vi "ToggleAqcuisitionRunning.vi"(8 "error in (no error)":errorcluster, 10 "Acquisition running":bool, 11 "ScopeBase In":refnum<class "ScopeBase.lvclass">) -> (0 "error out":errorcluster, 3 "ScopeBase Out":refnum<class "ScopeBase.lvclass">)   [LabVIEW 2025, in "ScopeBase.lvclass"]
uses:
  ScopeBase.lvclass
  ScopeBase.lvclass/ScopeBase.ctl
  <vilib>/Utility/error.llb/Error Cluster From Error Code.vi
  <vilib>/rvi/errors/niLvFpgaAdjustHostInterfaceError.vi
  <vilib>/rvi/interface/nirviReadWriteControl/nirviReadWriteControl.xnode
  FpgaRef/FpgaRefBase/Common FPGA ref.ctl
  FpgaRef/FpgaRefBase/FpgaRefBase.lvclass
  NiFpgaLv.dll
  <vilib>/rvi/interface/Simulation/niFpgaSimulationCallBeginRW.vi
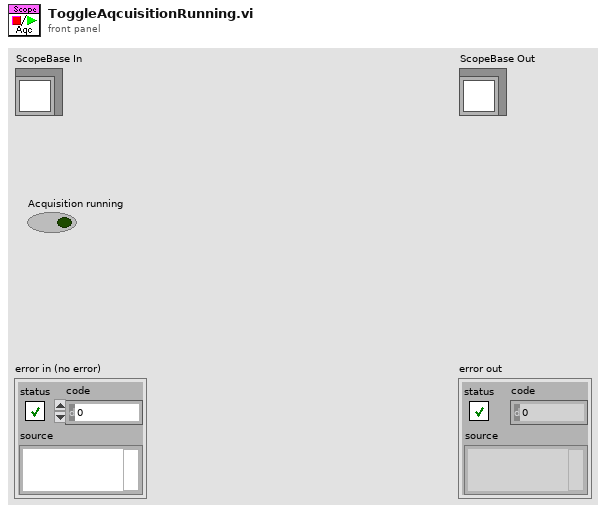
[diagram p1: front panel]
types:
  T1 = typedef "Common FPGA ref.ctl" = refnum<k20>
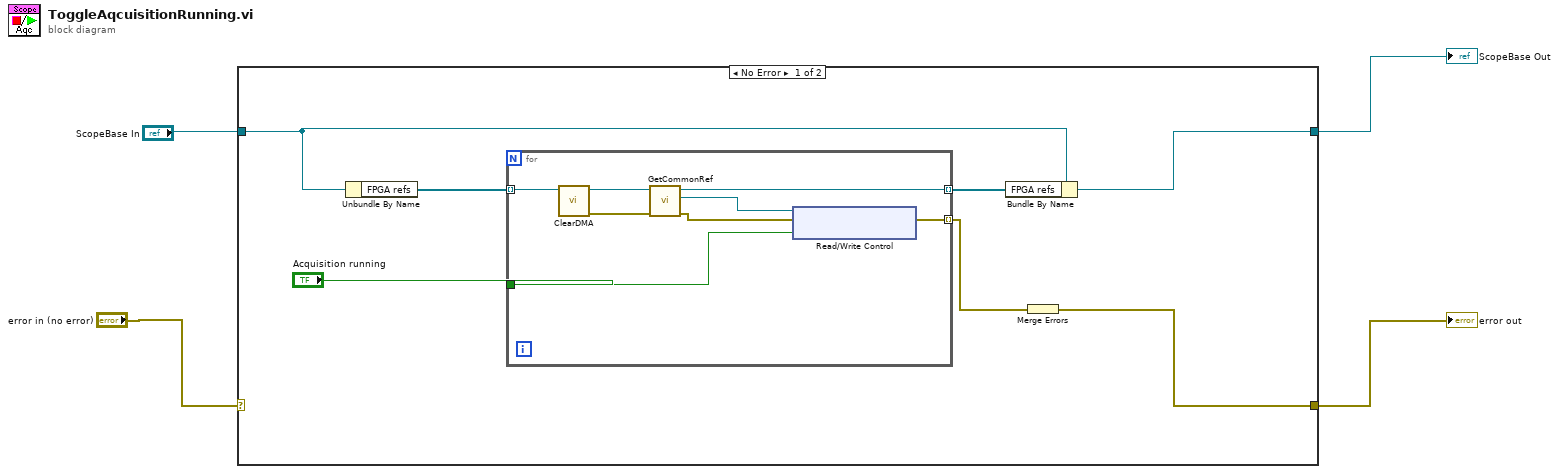
[diagram p0: block diagram]
diagram:
  n1 = case shown="No Error" "error in (no error)" {
    selector: "error in (no error)" -> [_ w21]
    tunnel: [w5 w21] -> w1
    tunnel: [w9 w20] -> w2
    tunnel: "ScopeBase In" -> [w7 w20]
    frame No Error {
      n2 = Unbundle By Name(w7) -> ("FPGA refs"=w11:refnum<class "FpgaRefBase.lvclass">[])
      n3 = for {
        tunnel: "Acquisition running" -> [w17]
        tunnel: w11 -> [w16] mode=indexing
        tunnel: [w19] -> w10 mode=indexing
        tunnel: [w14] -> w6 mode=indexing
        n4 = call-dynamic "ClearDMA.vi"("FpgaRefBase in"=w16) -> ("error out"=w13:errorcluster, "FpgaRefBase out"=w15:refnum<class "FpgaRefBase.lvclass">)  [unwired: 9 in]
        n5 = call-dynamic "GetCommonRef.vi"("error in (no error)"=w13, "FpgaRefBase in"=w15) -> ("error out"=w12:errorcluster, "Common ref"=w18:T1, "FpgaRefBase out"=w19:refnum<class "FpgaRefBase.lvclass">)  [unwired: 7 in]
        n6 = xnode "Read/Write Control"("FPGA VI Reference In"=w18, "error in"=w12, "Acquisition running"=w17) -> ("error out"=w14:errorcluster)  [unwired: 1 out]
      }
      n7 = Bundle By Name(cluster=w7, "FPGA refs"=w10) -> (w9:refnum<class "ScopeBase.lvclass">)
      n8 = Merge Errors(w6) -> (w5:errorcluster)
    }
    frame Error {
    }
  }
  "error out" <- w1
  "ScopeBase Out" <- w2
